vi "Find Record with Account.vi"(8 "error in (no error)":errorcluster, 10 "Account Number":dbl, 11 "Configuration Database in":refnum<class "ATM Controller.lvclass">) -> (0 "error out":errorcluster, 3 "Configuration Database out":refnum<class "ATM Controller.lvclass">)   [LabVIEW 2019]
uses:
  Configuration Database/Configuration Database Messages/Read Record Msg/Read Record Msg.lvclass
  ATM Controller.lvclass
  C:/Program Files (x86)/National Instruments/LabVIEW 2019/vi.lib/ActorFramework/Actor/Actor.lvclass
  <vilib>/ActorFramework/Message Enqueuer/Message Enqueuer.lvclass
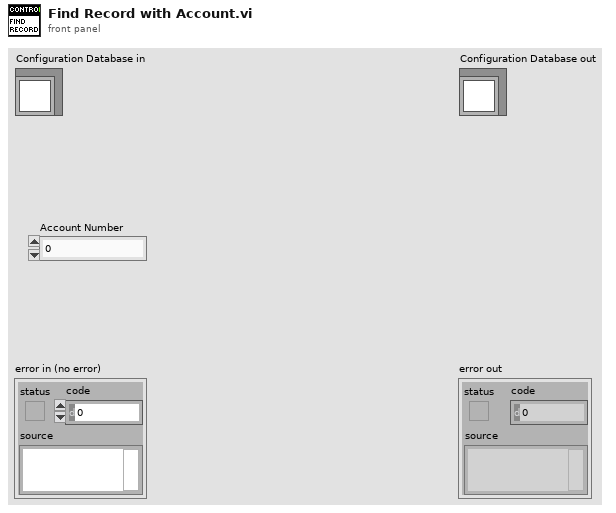
[diagram p1: front panel]
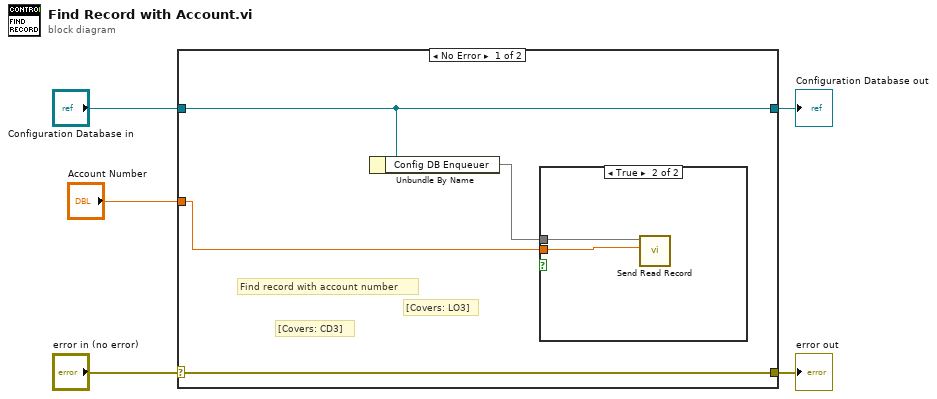
[diagram p0: block diagram]
diagram:
  n1 = case shown="No Error" "error in (no error)" {
    selector: "error in (no error)" -> [w9 w13]
    tunnel: [w9 w13] -> w4
    tunnel: [w8 w12] -> w2
    tunnel: "Configuration Database in" -> [w8 w12]
    tunnel: "Account Number" -> [w6 _]
    frame No Error {
      # "[Covers: LO3]"
      # "Find record with account number"
      # "[Covers: CD3]"
      n2 = Unbundle By Name(w8) -> ("Config DB Enqueuer"=w7)
      n3 = case shown="True" {
        selector: _ -> [_ _]
        tunnel: w7 -> [_ w11]
        tunnel: w6 -> [_ w10]
        frame False {
        }
        frame True {
          n4 = call "Send Read Record.vi"("Account Number"=w10, "Message Enqueuer"=w11) -> ()  [unwired: 8 in, 2 out]
        }
      }
    }
    frame Error {
    }
  }
  "error out" <- w4
  "Configuration Database out" <- w2
